vi "7 - DAQmx Bus Waveform Output and Input.vi"() -> ()   [LabVIEW 2021]
uses:
  <vilib>/TSA/Omni-Bus/Omni-Bus/Omni_Bus.lvclass
  <vilib>/TSA/Omni-Bus/Omni-Bus/Support/Broad Types.ctl
  <vilib>/Utility/Data Type/Type Definitions/Data Type.ctl
  <vilib>/TSA/Abstract Data Classes/Abs_Types/Type/Abs_Type.lvclass/Abs_Type.ctl
  <vilib>/TSA/Omni-Bus/Omni-Bus/Omni_Bus.lvclass/Omni_Bus.ctl
  <vilib>/TSA/Omni-Bus/Omni-Bus/Support/Read/Read Waveform.vi
  <vilib>/TSA/Omni-Bus/Omni-Bus/Support/Write/Write Waveform.vi
  <vilib>/TSA/Omni-Bus/Omni-Bus/Support/FindVar.vi
  <vilib>/Utility/error.llb/Clear Errors.vi
  <vilib>/TSA/Omni-Bus/Omni-Bus/Properties/Read Var Map.vi
  <vilib>/TSA/Abstract Data Classes/Abs_Types/Type/Properties/Read Tag.vi
  DAQmx-Bus.lvclass
  C:/Program Files (x86)/National Instruments/LabVIEW 2021/vi.lib/TSA/Omni-Bus/Omni-Bus/Bus Access/Bus_Access.lvclass
  <vilib>/TSA/Abstract Data Classes/Abs_Types/Waveform/Abs_Waveform.lvclass
  C:/Program Files (x86)/National Instruments/LabVIEW 2021/vi.lib/TSA/Abstract Data Classes/Abs_Types/Type/Abs_Type.lvclass
  <vilib>/TSA/Abstract Data Classes/Abs_Types/Value/Abs_Value.lvclass
  <vilib>/TSA/Omni-Bus/Omni-Bus/Support/Check For Read Only Error.vi
  <vilib>/TSA/Omni-Bus/Omni-Bus/Support/Incorrect Tag String Error.vi
  <vilib>/TSA/Abstract Data Classes/Abs_Types/Type/Abs_Type.lvclass
  <vilib>/measure/NI_MABase.lvlib
  <vilib>/Utility/Data Type/NI_Data Type.lvlib
panel:
  in  "DAQmx Task 2":refnum<k21>="VoltageWaveformOutput"
  in  "DAQmx Task 1":refnum<k21>="VoltageWaveformInput"
  in  "sampling info":cluster{"Fs":dbl, "#s":dbl}={"Fs"=1000.0, "#s"=1000.0} {"Fs" format="%.2p"}
  out "Waveform Chart":waveform(dbl)(graph)
  out "Stopping":bool
  in  "Waveform In Tag":string(combo)
  in  "amplitude":dbl=1.0 format="%0.2p"
  in  "signal type":T1(ring)
  in  "frequency":dbl=10.0 format="%0.2p"
  out "timed out?":bool
  in  "stop":bool
  in  "Waveform Out Tag":string(combo)
  # "Ouput Waveform"
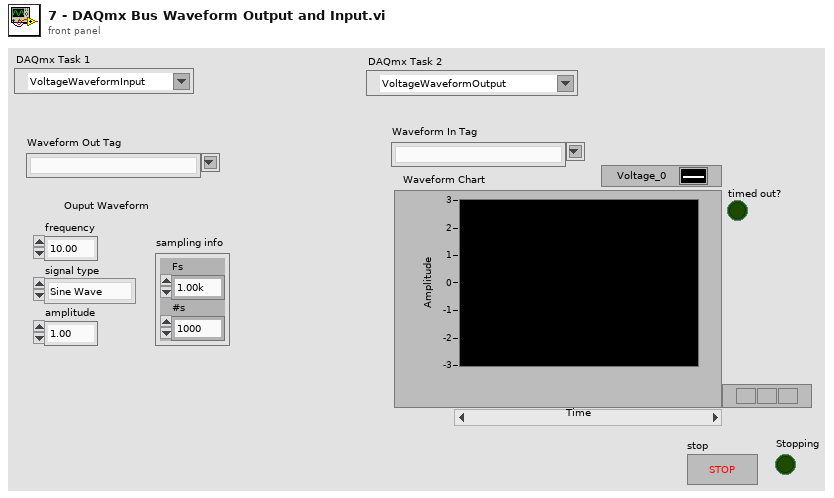
[diagram p1: front panel]
types:
  T1 = enum16{"Sine Wave", "Triangle Wave", "Square Wave", "Sawtooth Wave"}
  T2 = typedef "NI_Data Type.lvlib/Data Type.ctl" = enum8{"Invalid Type", "Void", "I8", "I16", "I32", "I64", "U8", "U16", "U32", "U64", "Single Float", "Double Float", "Extended Float", "Single Complex", "Double Complex", "Extended Complex", "Enum U8", "Enum U16", "Enum U32", "Enum U64", "Single Float With Unit", "Double Float With Unit", "Extended Float With Unit", "Single Complex with Unit", "Double Complex with Unit", "Extended Complex with Unit", "Boolean", "String", "Path", "Picture", "Tag", "Array", "Cluster", "Variant", "LV Variant", "Waveform", "Timestamp", "Digital Waveform", "Digital Data", "ExpressData", "Refnum", "External Data", "VI", "Poly VI", "LabVIEW Class Instance", "Fixed Point", "Set Collection", "Map Collection"}
  T3 = typedef "Omni_Bus.lvclass/Broad Types.ctl" = enum16{"All Tags", "NI Specific Type", "Boolean", "String", "Numeric", "Float", "Integer", "Collection", "All Value Types", "Non Value Types"}
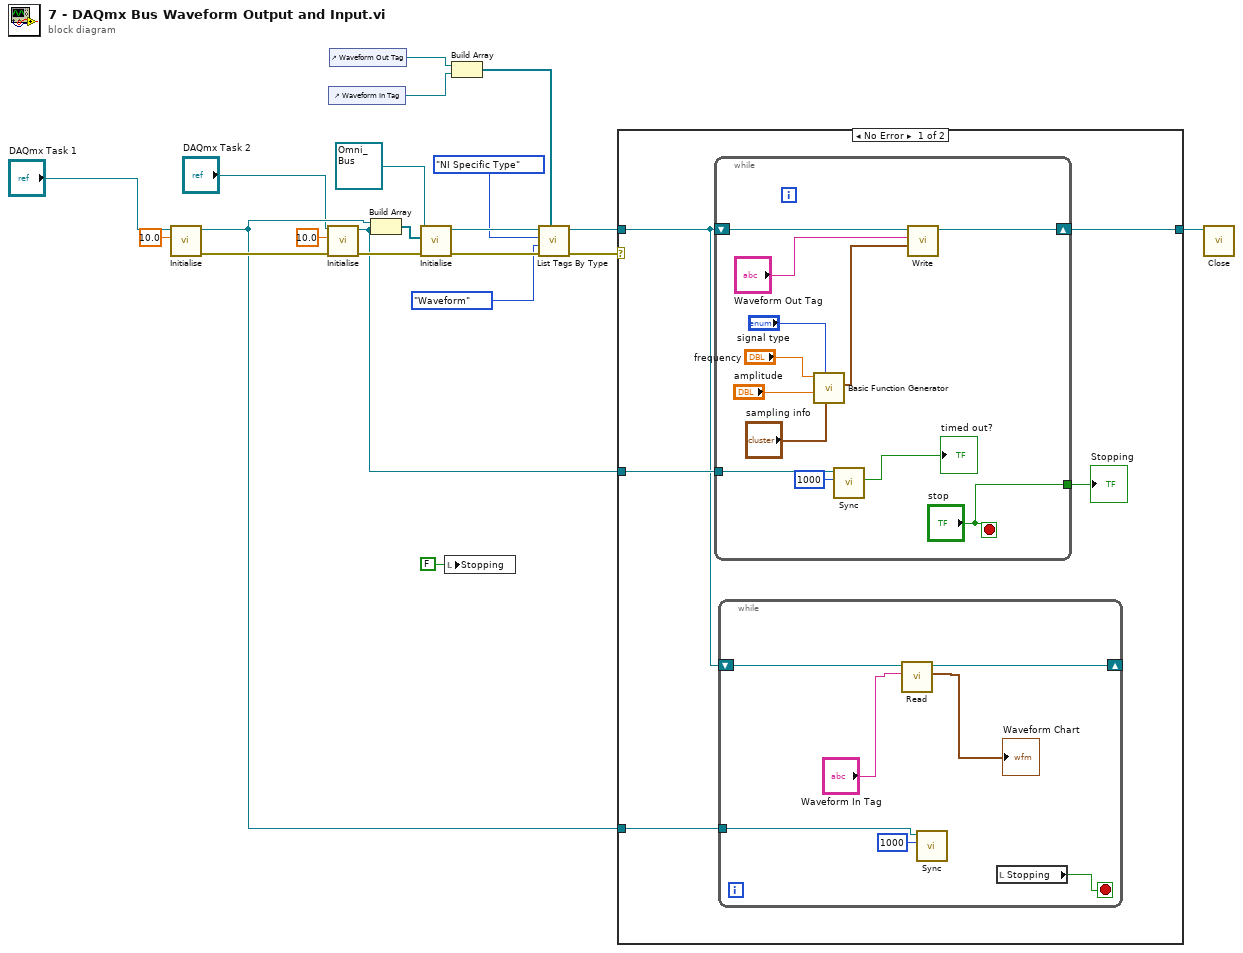
[diagram p0: block diagram]
diagram:
  n1 = call "Initialise.vi"("timeout (s)"=10.0 ("timeout"), "DAQmx Task"="DAQmx Task 1") -> ("error out"=w4:errorcluster, "DAQmx-Bus out"=w3:refnum<class "DAQmx-Bus.lvclass">)  [unwired: 8 in]
  n2 = call "Initialise.vi"("error in (no error)"=w4, "timeout (s)"=10.0 ("timeout"), "DAQmx Task"="DAQmx Task 2") -> ("error out"=w18:errorcluster, "DAQmx-Bus out"=w11:refnum<class "DAQmx-Bus.lvclass">)  [unwired: 7 in]
  n3 = control-ref of="Waveform In Tag"() -> (w8:refnum<vi>)
  n4 = control-ref of="Waveform Out Tag"() -> (w9:refnum<vi>)
  n5 = Build Array(w3, w11) -> (w20:refnum<class "DAQmx-Bus.lvclass">[])
  n6 = call-dynamic "Initialise.vi"("error in (no error)"=w18, "Bus Access"=w20, "Var Bus in"=refnum<class "Omni_Bus.lvclass"> refnum) -> ("error out"=w15:errorcluster, "Var Bus out"=w16:refnum<class "Omni_Bus.lvclass">)  [unwired: 7 in]
  n7 = local write "Stopping"(FALSE ("Stopping")) -> ()
  n8 = Build Array(w9, w8) -> (w7:refnum<vi>[])
  n9 = call <vilib>:"List Tags By Type.vi"("Combo Boxes"=w7, "error in (no error)"=w15, "NI Specific Type"=Data_Type."Waveform", "Broad Types"=Broad_Types."NI Specific Type", "Var Bus in"=w16) -> ("error out"=w13:errorcluster, "Var Bus out"=w14:refnum<class "Omni_Bus.lvclass">)  [unwired: 3 in, 2 out]
  n10 = case shown="No Error" w13 {
    tunnel: [w26 w46] -> w17
    tunnel: w14 -> [w24 w46]
    tunnel: w11 -> [w25 _]
    tunnel: w3 -> [w23 _]
    frame No Error {
      n11 = while {
        shift-right: [w36] -> w26
        shift-left: w24 -> [w45]
        tunnel: w25 -> [w43]
        tunnel: ["stop"] -> w22
        stop <- "stop" stop-if-true
        n12 = call <vilib>:"Basic Function Generator.vi"("sampling info"="sampling info", "signal type"="signal type", "amplitude"="amplitude", "frequency"="frequency") -> ("signal out"=w37:waveform(dbl))  [unwired: 5 in, 2 out]
        n13 = call-dynamic "Sync.vi"("timeout in ms (-1)"=1000, "DAQmx-Bus in"=w43) -> ("timed out?"=→"timed out?":bool)  [unwired: 7 in, 2 out]
        n14 = call-poly <vilib>:"Write.vi"("Waveform"=w37, "Tag"="Waveform Out Tag", "Omni_Bus in"=w45) -> ("Omni_Bus out"=w36:refnum<class "Omni_Bus.lvclass">)  [unwired: 7 in, 1 out]
      }
      "Stopping" <- w22
      n15 = while {
        shift-right: [w30] -> _
        shift-left: w24 -> [w31]
        tunnel: w23 -> [w29]
        stop <- w28 stop-if-true
        n16 = call-poly <vilib>:"Read.vi"("Tag"="Waveform In Tag", "Var Bus in"=w31) -> ("Waveform"=→"Waveform Chart":waveform(dbl), "Var Bus out"=w30:refnum<class "Omni_Bus.lvclass">)  [unwired: 7 in, 1 out]
        n17 = call-dynamic "Sync.vi"("timeout in ms (-1)"=1000, "DAQmx-Bus in"=w29) -> ()  [unwired: 7 in, 3 out]
        n18 = local read "Stopping"() -> (w28:bool)
      }
    }
    frame Error {
    }
  }
  n19 = call-dynamic "Close.vi"("Data in"=w17) -> ()  [unwired: 9 in, 2 out]
